vi "Data Queue.vi"(5 "timeout in ms (-1)":i32=10, 6 "max queue size (-1, unlimited)":i32, 7 "Action":T1=enum."Enqueue", 8 "error in (no error)":errorcluster, 11 "data in":u16[](array[numeric])) -> (0 "error out":errorcluster, 2 "# elements in queue":i32, 3 "data out":u16[](array[numeric]))   [LabVIEW 2018]
uses:
  Controls/Queue Manager Actions.ctl
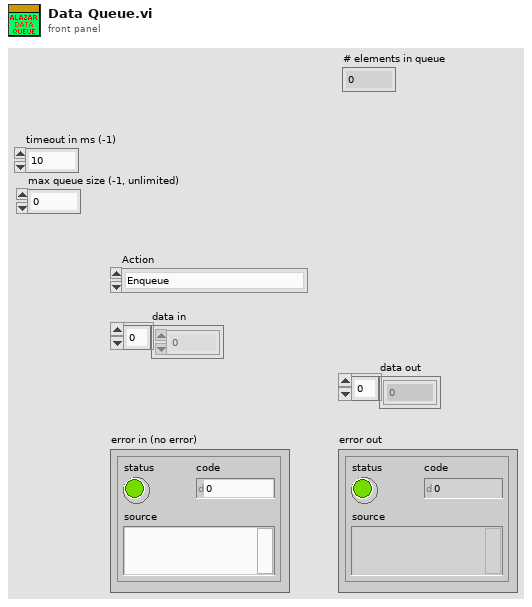
[diagram p1: front panel]
types:
  T1 = typedef "Queue Manager Actions.ctl" = enum16{"Init", "Enqueue", "Enqueue All", "Preview Queue", "Dequeue", "Get Status", "Flush Queue", "Flush All Queues", "Release All Queues", "Release Queue", "Enqueue at Opposite End"}
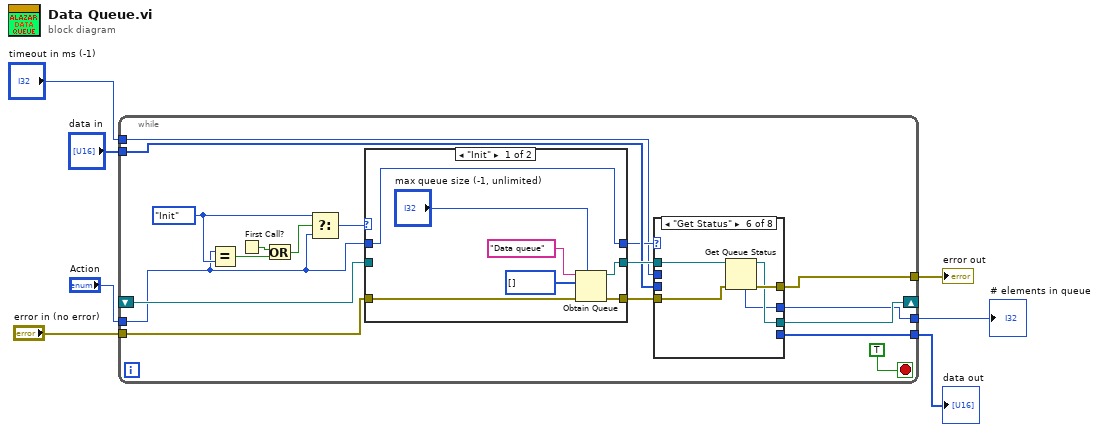
[diagram p0: block diagram]
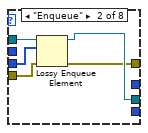
[diagram p3: hidden frame]
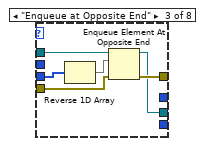
[diagram p4: hidden frame]
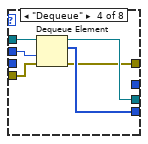
[diagram p5: hidden frame]
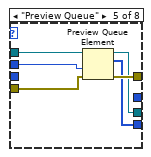
[diagram p6: hidden frame]
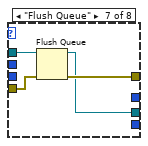
[diagram p7: hidden frame]
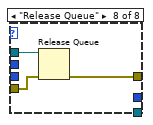
[diagram p8: hidden frame]
diagram:
  n1 = while {
    tunnel: "Action" -> [w10]
    tunnel: "error in (no error)" -> [w14]
    shift-right: [w16] -> _
    shift-left: _ -> [w15]
    tunnel: "data in" -> [w12]
    tunnel: "timeout in ms (-1)" -> [w9]
    tunnel: [w19] -> w3
    tunnel: [w18] -> w2
    tunnel: [w8] -> w1
    stop <- TRUE stop-if-true
    w21 = Queue_Manager_Actions."Init"
    n2 = Equal?(x=w10, y=w21) -> (x = y?=w23:bool)
    n3 = First Call?() -> (First Call?: T/F=w24:bool)
    n4 = Or(x=w24, y=w23) -> (x .or. y?=w22:bool)
    n5 = Select(t=w21, s=w22, f=w10) -> (s? t:f=w20:T1)
    n6 = case shown="\"Init\"" w20 {
      tunnel: [w69 w72] -> w17
      tunnel: [w68 w71] -> w13
      tunnel: w15 -> [_ w72]
      tunnel: w14 -> [w66 w71]
      tunnel: [w64 w70] -> w11
      tunnel: w10 -> [w64 w70]
      frame "Init" {
        n7 = Obtain Queue(max queue size (-1, unlimited)="max queue size (-1, unlimited)", name (unnamed)="Data queue", element data type=u16[] [], error in (no error)=w66) -> (queue out=w69:refnum<queue>, error out=w68:errorcluster)  [unwired: 1 in, 1 out]
      }
      frame Default {
      }
    }
    n8 = case shown="\"Get Status\"" w11 {
      tunnel: [w26 w28 w38 w39 w50 w55 w59 w62] -> w19
      tunnel: [_ _ _ w44 w49 _ _ _] -> w18
      tunnel: w17 -> [w27 w32 w35 w43 w47 w54 w58 w61]
      tunnel: [w27 w29 w36 w40 w46 w52 w56 _] -> w16
      tunnel: w13 -> [w26 w31 w34 w42 w48 w53 w57 w60]
      tunnel: w12 -> [_ w30 w33 _ _ _ _ _]
      tunnel: w9 -> [_ _ _ w41 w45 _ _ _]
      tunnel: [_ _ _ _ _ w51 _ _] -> w8
      frame "Init", Default {
      }
      frame "Enqueue" {
        n9 = Lossy Enqueue Element(queue=w32, element=w30, error in (no error)=w31) -> (queue out=w29:refnum<queue>, error out=w28:errorcluster)  [unwired: 2 out]
      }
      frame "Enqueue at Opposite End" {
        n10 = Reverse 1D Array(array=w33) -> (reversed array=w37:u16[])
        n11 = Enqueue Element At Opposite End(queue=w35, element=w37, error in (no error)=w34) -> (queue out=w36:refnum<queue>, error out=w38:errorcluster)  [unwired: 1 in, 1 out]
      }
      frame "Dequeue" {
        n12 = Dequeue Element(queue=w43, timeout in ms (-1)=w41, error in (no error)=w42) -> (queue out=w40:refnum<queue>, element=w44:u16[], error out=w39:errorcluster)  [unwired: 1 out]
      }
      frame "Preview Queue" {
        n13 = Preview Queue Element(queue=w47, timeout in ms (-1)=w45, error in (no error)=w48) -> (queue out=w46:refnum<queue>, element=w49:u16[], error out=w50:errorcluster)  [unwired: 1 out]
      }
      frame "Get Status" {
        n14 = Get Queue Status(queue=w54, error in (no error)=w53) -> (queue out=w52:refnum<queue>, error out=w55:errorcluster, # elements in queue=w51:i32)  [unwired: 1 in, 5 out]
      }
      frame "Flush Queue" {
        n15 = Flush Queue(queue=w58, error in (no error)=w57) -> (queue out=w56:refnum<queue>, error out=w59:errorcluster)  [unwired: 1 out]
      }
      frame "Release Queue" {
        n16 = Release Queue(queue=w61, error in (no error)=w60) -> (error out=w62:errorcluster)  [unwired: 1 in, 2 out]
      }
    }
  }
  "error out" <- w3
  "data out" <- w2
  "# elements in queue" <- w1
